vi "ComPortDialog.vi"(8 "error in (no error)":errorcluster caption="Fehler (Eingang - kein Fehler)", 9 "Com Port":i16=8 min=1, 10 "Com-Einst. in":T1={"COM"=1, "Baudrate"=enum."9600", "Echo"=TRUE, "Timeout"=200}, 11 "ini-File":path) -> (0 "error out":errorcluster caption="Fehler (Ausgang)", 2 "Com-Einst. out":T1={"COM"=0, "Baudrate"=enum."115200", "Echo"=FALSE, "Timeout"=200}, 3 "Abbruch":bool)   [LabVIEW 2014, in "K_S30c_dll.lvlib"]
uses:
  K_S30c_dll.lvlib
  <vilib>/Utility/config.llb/Read Key (Boolean).vi
  <vilib>/Utility/config.llb/Read Key (U32).vi
  <vilib>/Utility/config.llb/Read Key (I32).vi
  <vilib>/Utility/config.llb/Write Key (Boolean).vi
  <vilib>/Utility/config.llb/Write Key (I32).vi
  <vilib>/Utility/config.llb/NI_LVConfig.lvlib
panel:
  in  "Timeout":i16=200
  in  "Baudrate":enum16{"9600", "115200"}(ring)
  in  "Echo":bool
  in  "Enum":enum16{"wahl", "openCom", "weiter"}(ring)
  in  "cancel":bool
  # "Open Com Port"
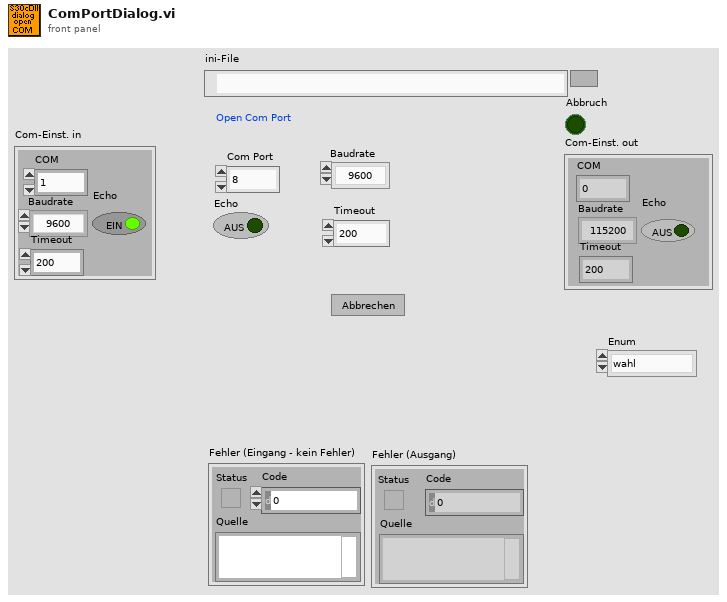
[diagram p1: front panel]
types:
  T1 = cluster{"COM":i16, "Baudrate":enum16{"9600", "115200"}, "Echo":bool, "Timeout":u32}
  T2 = typedef "NI_LVConfig.lvlib/Config Data RefNum.ctl" = refnum<k1>
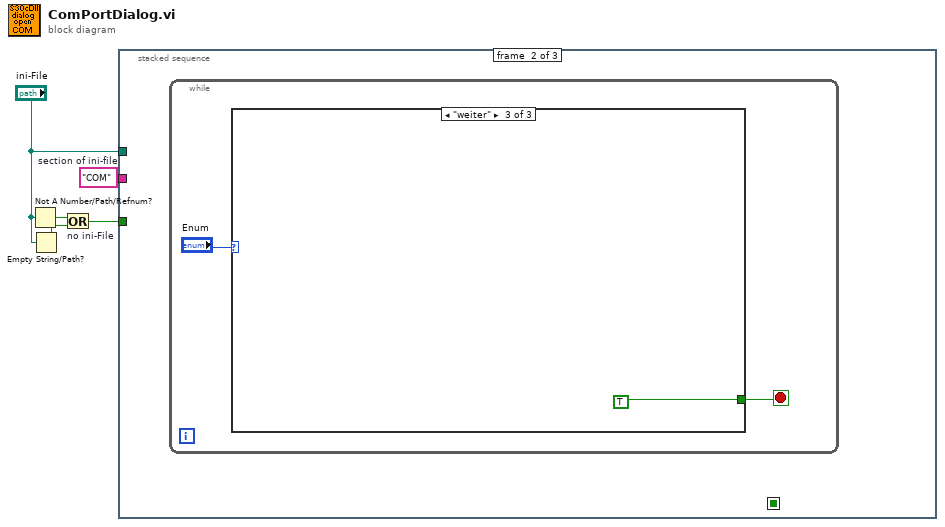
[diagram p0: block diagram]
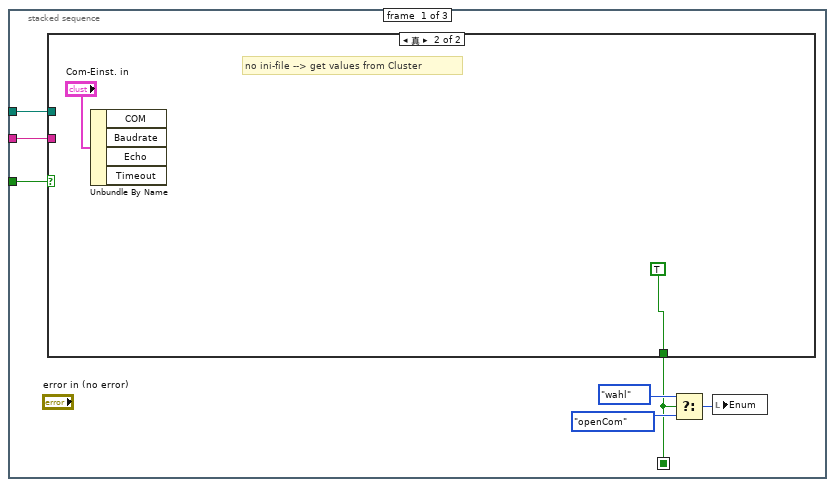
[diagram p2: hidden frame]
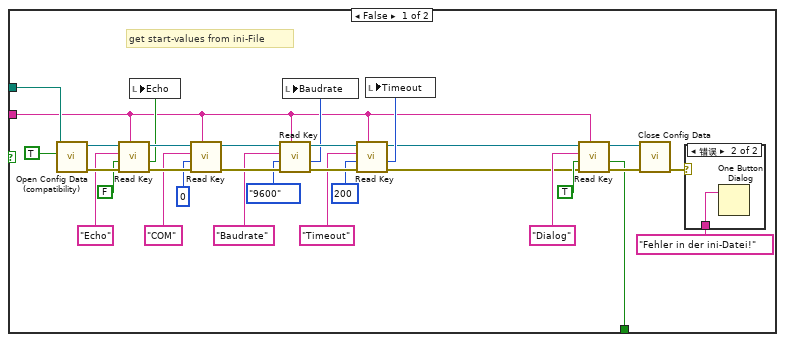
[diagram p3: hidden frame]
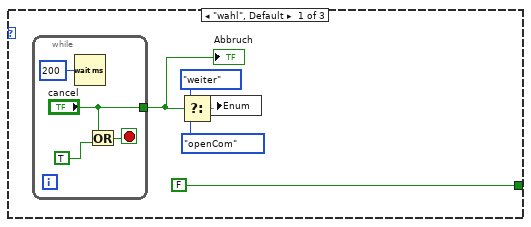
[diagram p5: hidden frame]
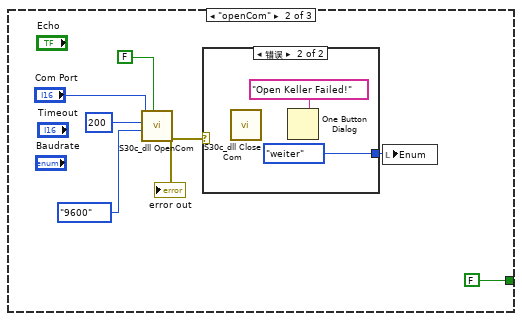
[diagram p6: hidden frame]
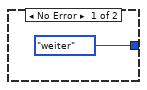
[diagram p7: hidden frame]
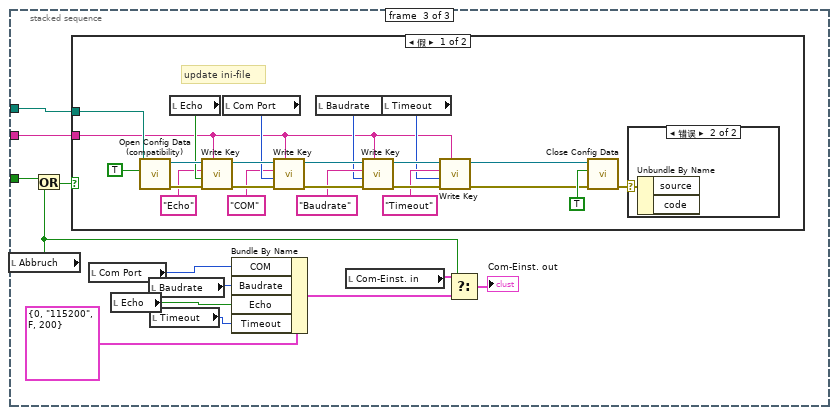
[diagram p8: hidden frame]
diagram:
  w1 = "COM"  # section of ini-file
  n1 = Not A Number/Path/Refnum?(number/path/refnum="ini-File") -> (NaN/Path/Refnum?=w5:bool)
  n2 = Empty String/Path?(string/path="ini-File") -> (empty?=w4:bool)
  n3 = Or "no ini-File"(x=w5, y=w4) -> (x .or. y?=w3:bool)
  n4 = stacked-sequence {
    seq-local: [w7 _ _] -> [_ _ _]
    tunnel: w3 -> [w12 _ w81]
    tunnel: "ini-File" -> [w11 _ w79]
    tunnel: w1 -> [w6 _ w69]
    frame #0 {
      n5 = case shown="真" w12 {
        tunnel: w11 -> [w43 _]
        tunnel: [w17 TRUE ("value")] -> w7
        tunnel: w6 -> [w13 _]
        frame False {
          # "get start-values from ini-File"
          n6 = call <vilib>:"Open Config Data (compatibility).vi"("create file if necessary (T)"=TRUE ("create file if necessary? (T)"), "configuration file path"=w43) -> ("error out"=w37:errorcluster, "refnum"=w41:T2)  [unwired: 7 in, 1 out]
          n7 = call-poly <vilib>:"Read Key.vi"("section"=w13, "error in (no error)"=w37, "default value"=FALSE, "key"="Echo", "refnum"=w41) -> ("error out"=w36:errorcluster, "value"=w30:bool, "refnum out"=w40:T2)  [unwired: 3 in, 1 out]
          n8 = local write "Echo"(w30) -> ()
          n9 = call-poly <vilib>:"Read Key.vi"("section"=w13, "error in (no error)"=w36, "default value"=u8 0, "key"="COM", "refnum"=w40) -> ("error out"=w35:errorcluster, "refnum out"=w39:T2)  [unwired: 3 in, 2 out]
          n10 = call-poly <vilib>:"Read Key.vi"("section"=w13, "error in (no error)"=w35, "default value"=enum16{"9600", "115200"}."9600", "key"="Baudrate", "refnum"=w39) -> ("error out"=w34:errorcluster, "value"=w25:i32, "refnum out"=w38:T2)  [unwired: 3 in, 1 out]
          n11 = local write "Baudrate"(w25) -> ()
          n12 = call-poly <vilib>:"Read Key.vi"("section"=w13, "error in (no error)"=w34, "default value"=u32 200, "key"="Timeout", "refnum"=w38) -> ("error out"=w15:errorcluster, "value"=w22:u32, "refnum out"=w14:T2)  [unwired: 3 in, 1 out]
          n13 = local write "Timeout"(w22) -> ()
          n14 = call-poly <vilib>:"Read Key.vi"("section"=w13, "error in (no error)"=w15, "default value"=TRUE, "key"="Dialog", "refnum"=w14) -> ("error out"=w19:errorcluster, "value"=w17:bool, "refnum out"=w18:T2)  [unwired: 3 in, 1 out]
          n15 = call <vilib>:"Close Config Data.vi"("error in (no error)"=w19, "refnum"=w18) -> ("error out"=w24:errorcluster)  [unwired: 8 in, 1 out]
          n16 = case shown="错误" w24 {
            tunnel: "Fehler in der ini-Datei!" ("Nachricht") -> [_ w44]
            frame No Error {
            }
            frame Error {
              n17 = One Button Dialog(message=w44) -> ()  [unwired: 1 in, 1 out]
            }
          }
        }
        frame True {
          # "no ini-file --> get values from Cluster"
          n18 = Unbundle By Name("Com-Einst. in") -> ()  [unwired: 4 out]
        }
      }
      n19 = Select(t=enum16{"wahl", "openCom", "weiter"}."wahl" ("Enum"), s=w7, f=enum16{"wahl", "openCom", "weiter"}."openCom" ("Enum")) -> (s? t:f=w10:enum16{"wahl", "openCom", "weiter"})
      n20 = local write "Enum"(w10) -> ()
    }
    frame #1 {
      n21 = while {
        stop <- w47 stop-if-true
        n22 = case shown="\"weiter\"" "Enum" {
          tunnel: [FALSE FALSE TRUE] -> w47
          frame "wahl", Default {
            n23 = while {
              tunnel: ["cancel"] -> w52
              stop <- w56 stop-if-true
              n24 = Wait (ms)(milliseconds to wait=u32 200 ("Zu wartende ms")) -> ()  [unwired: 1 out]
              n25 = Or(x="cancel", y=TRUE ("ok")) -> (x .or. y?=w56:bool)
            }
            "Abbruch" <- w52
            n26 = Select(t=enum16{"wahl", "openCom", "weiter"}."weiter" ("Enum"), s=w52, f=enum16{"wahl", "openCom", "weiter"}."openCom" ("Enum")) -> (s? t:f=w51:enum16{"wahl", "openCom", "weiter"})
            n27 = local write "Enum"(w51) -> ()
          }
          frame "openCom" {
            n28 = call "S30c_dll OpenCom.vi"("Echo (RS485 converter)"=FALSE ("Echo"), "Baudrate"=enum16{"9600", "115200"}."9600", "Timeout"=i16 200, "ComPort-Nr."="Com Port") -> ("error out"=w62:errorcluster)  [unwired: 5 in]
            "error out" <- w62
            n29 = case shown="错误" w62 {
              tunnel: [enum16{"wahl", "openCom", "weiter"}."weiter" ("Enum") enum16{"wahl", "openCom", "weiter"}."weiter" ("Enum")] -> w64
              frame No Error {
              }
              frame Error {
                n30 = call "S30c_dll Close Com.vi"() -> ()  [unwired: 7 in, 1 out]
                n31 = One Button Dialog(message="Open Keller Failed!" ("Nachricht")) -> ()  [unwired: 1 in, 1 out]
              }
            }
            n32 = local write "Enum"(w64) -> ()
          }
          frame "weiter" {
          }
        }
      }
    }
    frame #2 {
      n33 = local read "Abbruch"() -> (w78:bool)
      n34 = Or(x=w81, y=w78) -> (x .or. y?=w80:bool)
      n35 = case shown="假" w80 {
        tunnel: w79 -> [w86 _]
        tunnel: w69 -> [w82 _]
        frame False {
          # "update ini-file"
          n36 = call <vilib>:"Open Config Data (compatibility).vi"("create file if necessary (T)"=TRUE ("create file if necessary? (T)"), "configuration file path"=w86) -> ("error out"=w99:errorcluster, "refnum"=w103:T2)  [unwired: 7 in, 1 out]
          n37 = local read "Echo"() -> (w95:bool)
          n38 = call-poly <vilib>:"Write Key.vi"("section"=w82, "error in (no error)"=w99, "value"=w95, "key"="Echo", "refnum"=w103) -> ("error out"=w98:errorcluster, "refnum out"=w102:T2)  [unwired: 4 in, 1 out]
          n39 = local read "Com Port"() -> (w94:i16)
          n40 = call-poly <vilib>:"Write Key.vi"("section"=w82, "error in (no error)"=w98, "value"=w94, "key"="COM", "refnum"=w102) -> ("error out"=w97:errorcluster, "refnum out"=w101:T2)  [unwired: 4 in, 1 out]
          n41 = local read "Baudrate"() -> (w89:enum16{"9600", "115200"})
          n42 = call-poly <vilib>:"Write Key.vi"("section"=w82, "error in (no error)"=w97, "value"=w89, "key"="Baudrate", "refnum"=w101) -> ("error out"=w96:errorcluster, "refnum out"=w100:T2)  [unwired: 4 in, 1 out]
          n43 = local read "Timeout"() -> (w85:i16)
          n44 = call-poly <vilib>:"Write Key.vi"("section"=w82, "error in (no error)"=w96, "value"=w85, "key"="Timeout", "refnum"=w100) -> ("error out"=w84:errorcluster, "refnum out"=w83:T2)  [unwired: 4 in, 1 out]
          n45 = call <vilib>:"Close Config Data.vi"("error in (no error)"=w84, "write file if changed (T)"=TRUE ("write configuration file? (T)"), "refnum"=w83) -> ("error out"=w88:errorcluster)  [unwired: 7 in, 1 out]
          n46 = case shown="错误" w88 {
            selector: w88 -> [_ w105]
            frame No Error {
            }
            frame Error {
              n47 = Unbundle By Name(w105) -> ()  [unwired: 2 out]
            }
          }
        }
        frame True {
          # "no ini-file or cancel --> don't change the  ini file"
        }
      }
      n48 = local read "Com Port"() -> (w74:i16)
      n49 = local read "Echo"() -> (w72:bool)
      n50 = local read "Baudrate"() -> (w73:enum16{"9600", "115200"})
      n51 = local read "Timeout"() -> (w71:i16)
      n52 = Bundle By Name(cluster=T1 {"COM"=0, "Baudrate"=enum."115200", "Echo"=FALSE, "Timeout"=200} ("Com-Einst. out"), "COM"=w74, "Baudrate"=w73, "Echo"=w72, "Timeout"=w71) -> (w70:T1)
      n53 = local read "Com-Einst. in"() -> (w76:T1)
      n54 = Select(t=w76, s=w78, f=w70) -> (s? t:f=→"Com-Einst. out":T1)
    }
  }
